vi "HMI Pop Up Alpha KB.vi"(4 "Password Display (F)":bool, 5 "Hide Insert Key (T)":bool, 6 "Max Length (70)":u32=70, 10 "String In":string="13182713", 11 "Message In":string="Customer Part No.") -> (1 "Canceled":bool=TRUE, 2 "String Out":string="13182713")   [LabVIEW 2018]
doc: "Name: Pop Up Keyboard\nAuthor: Georges Janveau, Columbia Forest Products\nCreated:6/10/05\n\nDESCRIPTION\nSimulates an alphanumeric keyboard intended to be used on a touchscreen PC. The input control can be set for standard or password display. The OVR key can be shown or hidden.\n\nINPUTS\nMessage In - Optional message displayedin the title bar.\nString In - Sets the initial value of the edit box.\nPassword Display (F) - Sets standard or password display.\nHide OVR Key (T) - Hides or displays the OVR key button.\nMax Length (255) - Sets the maximum length allowed in the edit box.\n\nOUTPUTS\nString Out - Result (will contain String In if the user cancels).\nCanceled - True if the user cancels.\n\n----------------------------------------------------------------------------------------------------------------"
panel:
  in  "Clear":bool
  out "Caps on":bool
  in  "Shift 2":bool
  in  "<\n,":bool
  in  "?\n/":bool
  in  ">\n.":bool
  in  "M\nm":bool
  in  "N\nn":bool
  in  "B\nb":bool
  in  "V\nv":bool
  in  "C\nc":bool
  in  "X\nx":bool
  in  "Y\ny":bool
  in  "\"\n'":bool
  in  ":\n;":bool
  in  "L\nl":bool
  in  "K\nk":bool
  in  "J\nj":bool
  in  "H\nh":bool
  in  "G\ng":bool
  in  "F\nf":bool
  in  "D\nd":bool
  in  "S\ns":bool
  in  "A\na":bool
  in  "}\n]":bool
  in  "{\n[":bool
  in  "|\n\\":bool
  in  "+\n=":bool
  in  "_\n-":bool
  in  "P\np":bool
  in  "O\no":bool
  in  "I\ni":bool
  in  "U\nu":bool
  in  "Z\nz":bool
  in  "T\nt":bool
  in  "R\nr":bool
  in  "E\ne":bool
  in  "W\nw":bool
  in  ")\n0":bool
  in  "(\n9":bool
  in  "*\n8":bool
  in  "&\n7":bool
  in  "^\n6":bool
  in  "%\n5":bool
  in  "$\n4":bool
  in  "#\n3":bool
  in  "@\n2":bool
  in  "!\n1":bool
  in  "Q\nq":bool
  in  "Right":bool
  in  "Left":bool
  in  "Insert Overlay":bool
  in  "Enter":bool
  in  "Esc":bool
  in  "Space":bool
  in  "Shift":bool
  in  "CAPS":bool
  in  "Text":string
  in  "Backspace":bool
  # "Inputs"
  # "Outputs"
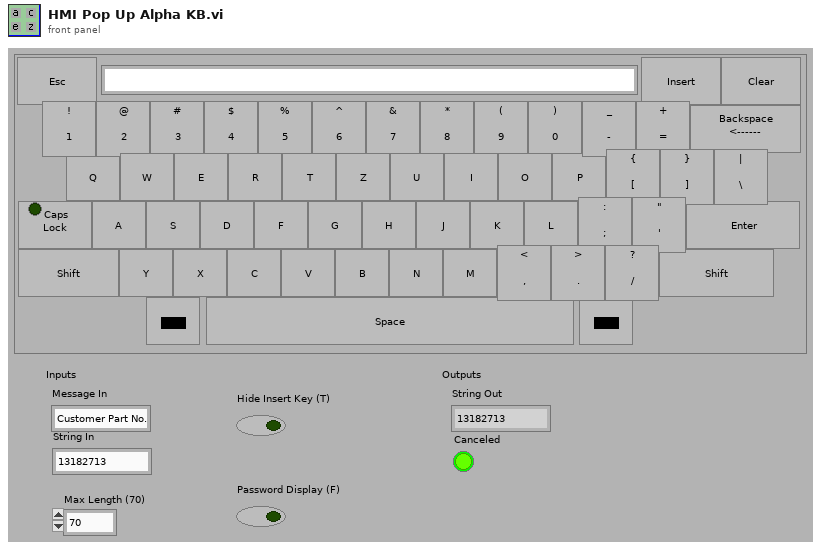
[diagram p1: front panel]
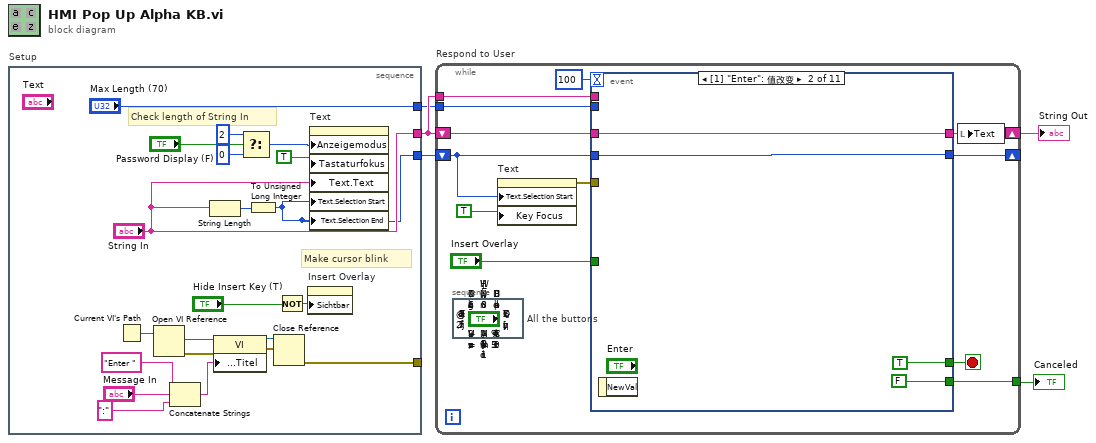
[diagram p0: block diagram]
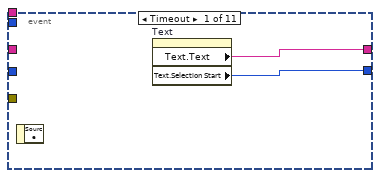
[diagram p2: hidden frame]
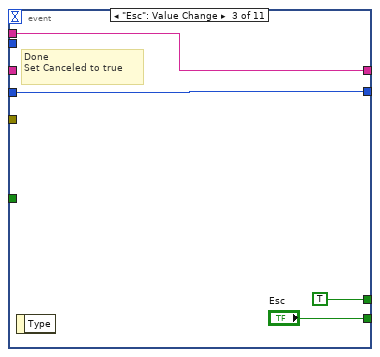
[diagram p3: hidden frame]
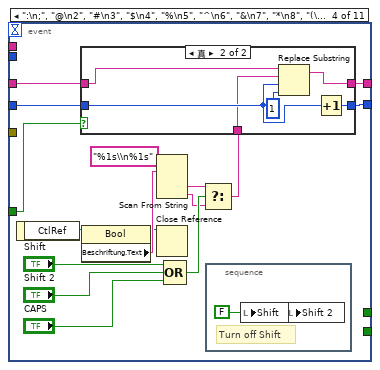
[diagram p4: hidden frame]
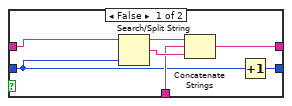
[diagram p5: hidden frame]
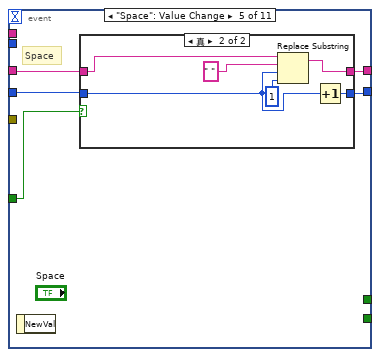
[diagram p6: hidden frame]
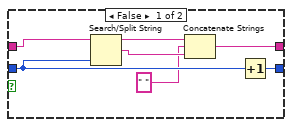
[diagram p7: hidden frame]
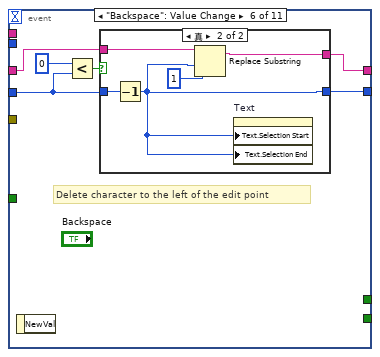
[diagram p8: hidden frame]
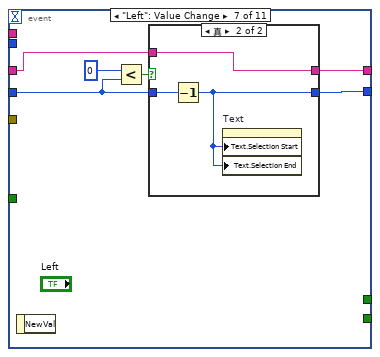
[diagram p10: hidden frame]
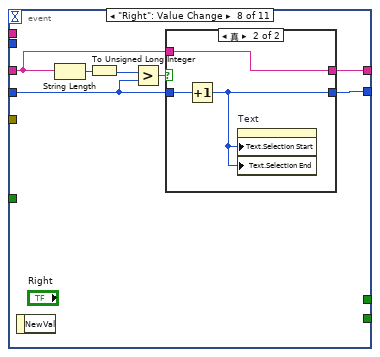
[diagram p12: hidden frame]
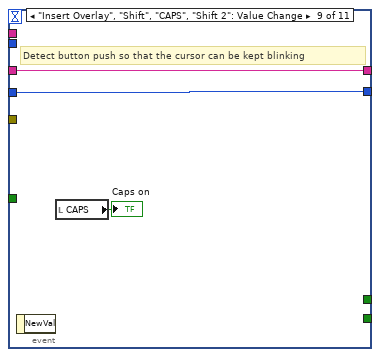
[diagram p14: hidden frame]
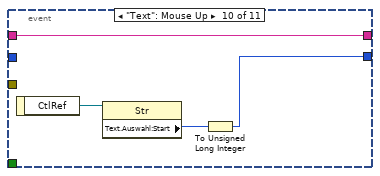
[diagram p15: hidden frame]
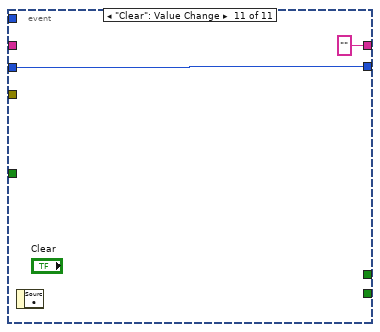
[diagram p16: hidden frame]
diagram:
  n1 = stacked-sequence "Setup" {
    tunnel: ["String In"] -> w3
    tunnel: [w10] -> _
    tunnel: ["Max Length (70)"] -> w2
    tunnel: [w6] -> w1
    frame #0 {
      # "Check length of String In"
      # "Make cursor blink"
      n2 = Current VI's Path() -> (path=w13:path)
      n3 = Open VI Reference(vi path=w13) -> (vi reference=w14:refnum<vi>, error out=w15:errorcluster)  [unwired: 1 in, 4 out]
      n4 = Concatenate Strings("Enter ", "Message In", ":" ("Substring")) -> (w18:string)
      n5 = String Length(string="String In") -> (length=w9:i32)
      n6 = property class="VI"(reference=w14, error in=w15, "Frontpanel-Fenster:Titel"=w18) -> (reference out=w16:refnum<vi>, error out=w17:errorcluster)
      n7 = Select(t=u32 2 ("Display Style"), s="Password Display (F)", f=u32 0 ("Display Style")) -> (s? t:f=w22:u32)
      n8 = To Unsigned Long Integer(number=w9) -> (unsigned 32bit integer=w6:u32)
      n9 = Close Reference(reference=w16, error in (no error)=w17) -> (error out=w10:errorcluster)
      n10 = Not(x="Hide Insert Key (T)") -> (.not. x?=w19:bool)
      n11 = property on="Insert Overlay" class="Bool (严格)"("Sichtbar"=w19) -> ()  [unwired: 2 in, 2 out]
      n12 = property on="Text" class="Str"("Anzeigemodus"=w22, "Tastaturfokus"=TRUE ("Key Focus"), "Text.Text"="String In", "Text.Selection Start"=w6, "Text.Selection End"=w6) -> ()  [unwired: 2 in, 2 out]
    }
  }
  n13 = while "Respond to User" {
    tunnel: [w37] -> w5
    tunnel: w3 -> [w36]
    shift-right: [w29] -> w4
    shift-left: w3 -> [w33]
    tunnel: w2 -> [w34]
    shift-right: [w31] -> _
    shift-left: w1 -> [w27]
    stop <- w38 stop-if-true
    n14 = stacked-sequence "All the buttons" {
      frame #0 {
      }
    }
    n15 = property on="Text" class="Str"("Text.Selection Start"=w27, "Key Focus"=TRUE) -> (error out=w28:errorcluster)  [unwired: 2 in, 1 out]
    n16 = event shown="[1] \"Enter\": 值改变" {
      selector: _ -> [_ _ _ _ _ _ _ _ _ _ _]
      dyn-events: _ -> [_ _ _ _ _ _ _ _ _ _ _]
      timeout: 100 -> [_ _ _ _ _ _ _ _ _ _ _]
      tunnel: [_ TRUE TRUE _ _ _ _ _ _ _ _] -> w38
      tunnel: [_ FALSE ("Cancel") "Esc" _ _ _ _ _ _ _ _] -> w37
      tunnel: w33 -> [_ w42 _ w52 w80 w100 w113 w121 w134 w136 _]
      tunnel: [w40 w42 w46 w49 w83 w99 w112 w122 w134 w136 ""] -> w29
      tunnel: w36 -> [_ _ w46 _ _ _ _ _ _ _ _]
      tunnel: "Insert Overlay" -> [_ _ _ w54 w81 _ _ _ _ _ _]
      tunnel: w34 -> [_ _ _ _ _ _ _ _ _ _ _]
      tunnel: w27 -> [_ w41 w45 w51 w79 w98 w110 w124 w133 _ w141]
      tunnel: [w39 w41 w45 w50 w82 w97 w111 w123 w133 w137 w141] -> w31
      tunnel: w28 -> [_ _ _ _ _ _ _ _ _ _ _]
      event Timeout {
        n17 = event-data() -> ()  [unwired: 2 out]
        n18 = property on="Text" class="Str"() -> ("Text.Text"=w40:string, "Text.Selection Start"=w39:u32)  [unwired: 2 in, 2 out]
      }
      event "Enter": Value Change {
        n19 = event-data() -> ()  [unwired: 2 out]
      }
      event "Esc": Value Change {
        # "Done\nSet Canceled to true"
        n20 = event-data() -> ()  [unwired: 2 out]
      }
      event ":\n;", "@\n2", "#\n3", "$\n4", "%\n5", "^\n6", "&\n7", "*\n8", "(\n9", ")\n0", "_\n-", "+\n=", "|\n\\", "Q\nq", "W\nw", "E\ne", "R\nr", "T\nt", "Z\nz", "U\nu", "I\ni", "O\no", "P\np", "A\na", "S\ns", "D\nd", "F\nf", "G\ng", "H\nh", "J\nj", "K\nk", "L\nl", "\"\n'", "Y\ny", "X\nx", "C\nc", "V\nv", "B\nb", "N\nn", "M\nm", "<\n,", ">\n.", "?\n/", "}\n]", "!\n1": Value Change {
        n21 = event-data() -> ("CtlRef"=w60:refnum<vi>)  [unwired: 1 out]
        n22 = property class="Bool"(reference=w60) -> (reference out=w58:refnum<vi>, "Beschriftung.Text"=w59:string)  [unwired: 1 in, 1 out]
        n23 = Scan From String(format string="%1s\\n%1s", input string=w59) -> (output 1=w62:string, output 2=w61:string)  [unwired: 2 in, 5 out]
        n24 = Close Reference(reference=w58) -> ()  [unwired: 1 in, 1 out]
        n25 = Compound Arithmetic op=OR("Shift", "Shift 2", "CAPS") -> (w63:bool)
        n26 = Select(t=w62, s=w63, f=w61) -> (s? t:f=w53:string)
        n27 = case shown="真" w54 {
          tunnel: w53 -> [w70 w73]
          tunnel: w52 -> [w69 w78]
          tunnel: w51 -> [w68 w76]
          tunnel: [w67 w77] -> w50
          tunnel: [w66 w74] -> w49
          frame False {
            n28 = Search/Split String(string=w69, offset (0)=w68) -> (substring before match=w72:string, match + rest of string=w71:string)  [unwired: 2 out]
            n29 = Concatenate Strings(w72, w70, w71) -> (w66:string)
            n30 = Increment(x=w68) -> (x+1=w67:u32)
          }
          frame True {
            n31 = Replace Substring(2:1, 3:w76, 4:w73, 5:w78) -> (1:w74:string)  [unwired: 1 out]
            n32 = Increment(x=w76) -> (x+1=w77:u32)
          }
        }
        n33 = stacked-sequence {
          frame #0 {
            w65 = FALSE ("Shift")
            # "Turn off Shift"
            n34 = local write "Shift"(w65) -> ()
            n35 = local write "Shift 2"(w65) -> ()
          }
        }
      }
      event "Space": Value Change {
        # "Space"
        n36 = event-data() -> ()  [unwired: 2 out]
        n37 = case shown="真" w81 {
          tunnel: w80 -> [w88 w96]
          tunnel: w79 -> [w87 w94]
          tunnel: [w86 w95] -> w82
          tunnel: [w85 w92] -> w83
          frame False {
            n38 = Search/Split String(string=w88, offset (0)=w87) -> (substring before match=w90:string, match + rest of string=w89:string)  [unwired: 2 out]
            n39 = Concatenate Strings(w90, " ", w89) -> (w85:string)
            n40 = Increment(x=w87) -> (x+1=w86:u32)
          }
          frame True {
            n41 = Replace Substring(2:1, 3:w94, 4:" ", 5:w96) -> (1:w92:string)  [unwired: 1 out]
            n42 = Increment(x=w94) -> (x+1=w95:u32)
          }
        }
      }
      event "Backspace": Value Change {
        # "Delete character to the left of the edit point"
        n43 = event-data() -> ()  [unwired: 2 out]
        n44 = Less?(x=u32 0, y=w98) -> (x < y?=w101:bool)
        n45 = case shown="真" w101 {
          tunnel: w100 -> [w104 w109]
          tunnel: w98 -> [w103 w107]
          tunnel: [w103 w105] -> w97
          tunnel: [w104 w106] -> w99
          frame False {
          }
          frame True {
            n46 = Decrement(x=w107) -> (x-1=w105:u32)
            n47 = Replace Substring(2:1, 3:w105, 5:w109) -> (1:w106:string)  [unwired: 2 out]
            n48 = property on="Text" class="Str"("Text.Selection Start"=w105, "Text.Selection End"=w105) -> ()  [unwired: 2 in, 2 out]
          }
        }
      }
      event "Left": Value Change {
        n49 = event-data() -> ()  [unwired: 2 out]
        n50 = Less?(x=u32 0, y=w110) -> (x < y?=w115:bool)
        n51 = case shown="真" w115 {
          tunnel: w113 -> [w117 w119]
          tunnel: w110 -> [w116 w120]
          tunnel: [w116 w118] -> w111
          tunnel: [w117 w119] -> w112
          frame False {
          }
          frame True {
            n52 = Decrement(x=w120) -> (x-1=w118:u32)
            n53 = property on="Text" class="Str"("Text.Selection Start"=w118, "Text.Selection End"=w118) -> ()  [unwired: 2 in, 2 out]
          }
        }
      }
      event "Right": Value Change {
        n54 = event-data() -> ()  [unwired: 2 out]
        n55 = String Length(string=w121) -> (length=w125:i32)
        n56 = To Unsigned Long Integer(number=w125) -> (unsigned 32bit integer=w126:u32)
        n57 = Greater?(x=w126, y=w124) -> (0:w127:bool)
        n58 = case shown="真" w127 {
          tunnel: w121 -> [w129 w131]
          tunnel: w124 -> [w128 w132]
          tunnel: [w128 w130] -> w123
          tunnel: [w129 w131] -> w122
          frame False {
          }
          frame True {
            n59 = Increment(x=w132) -> (x+1=w130:u32)
            n60 = property on="Text" class="Str"("Text.Selection Start"=w130, "Text.Selection End"=w130) -> ()  [unwired: 2 in, 2 out]
          }
        }
      }
      event "Insert Overlay", "Shift", "CAPS", "Shift 2": Value Change {
        # "Detect button push so that the cursor can be kept blinking"
        n61 = event-data() -> ()  [unwired: 2 out]
        n62 = local read "CAPS"() -> (→"Caps on":bool)
      }
      event "Text": Mouse Up {
        n63 = event-data() -> ("CtlRef"=w138:refnum<vi>)  [unwired: 1 out]
        n64 = property class="Str"(reference=w138) -> ("Text.Auswahl:Start"=w139:u32)  [unwired: 1 in, 2 out]
        n65 = To Unsigned Long Integer(number=w139) -> (unsigned 32bit integer=w137:u32)
      }
      event "Clear": Value Change {
        n66 = event-data() -> ()  [unwired: 2 out]
      }
    }
    n67 = local write "Text"(w29) -> ()
  }
  "Canceled" <- w5
  "String Out" <- w4
